vi "OPC Query.vi"(8 "error in (no error)":errorcluster, 11 "VISA resource name":refnum<visa-resource-name>) -> (0 "error out":errorcluster, 2 "*OPC? returns":i16, 3 "VISA resource name out":refnum<visa-resource-name>)   [LabVIEW 2020, in "ADCMT7451_ADC.lvlib"]
doc: "Send *OPC? command and receive response."
uses:
  ADCMT7451_ADC.lvlib
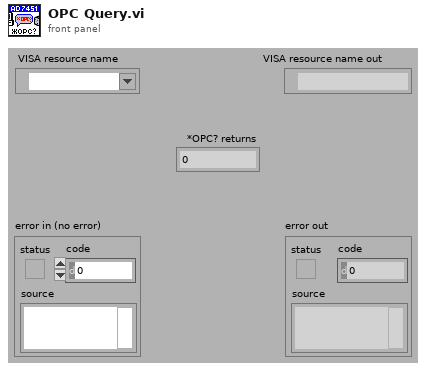
[diagram p1: front panel]
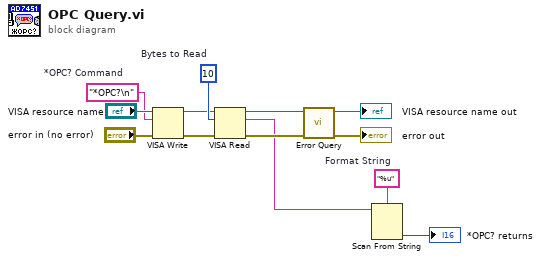
[diagram p0: block diagram]
diagram:
  w3 = "%u"  # Format String
  w9 = "*OPC?\n"  # *OPC? Command
  w12 = u32 10  # Bytes to Read
  n1 = VISA Write(VISA resource name="VISA resource name", write buffer=w9, error in (no error)="error in (no error)") -> (VISA resource name out=w11:refnum<visa-resource-name>, error out=w10:errorcluster)  [unwired: 1 out]
  n2 = VISA Read(VISA resource name=w11, byte count=w12, error in (no error)=w10) -> (VISA resource name out=w7:refnum<visa-resource-name>, read buffer=w1:string, error out=w8:errorcluster)  [unwired: 1 out]
  n3 = call "Error Query.vi"("error in (no error)"=w8, "VISA resource name"=w7) -> ("error out"=→"error out":errorcluster, "VISA resource name out"=→"VISA resource name out":refnum<visa-resource-name>)  [unwired: 6 in, 2 out]
  n4 = Scan From String(format string=w3, input string=w1) -> (output 1=→"*OPC? returns":i16)  [unwired: 3 in, 3 out]
